vi "FindDeviceNumber.vi"(11 "device":string) -> (3 "device":u16)   [LabVIEW 2022 SP3]
uses:
  Mic/Mic_Global.vi
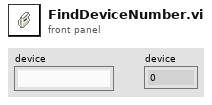
[diagram p1: front panel]
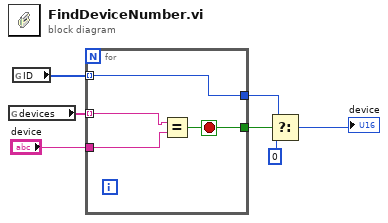
[diagram p0: block diagram]
diagram:
  n1 = global read "Mic_Global.vi" "devices"() -> (w7:string[])
  n2 = global read "Mic_Global.vi" "ID"() -> (w1:i32[])
  n3 = for {
    tunnel: w7 -> [w9] mode=indexing
    tunnel: "device" -> [w11]
    tunnel: [w8] -> w4
    tunnel: [w10] -> w5
    tunnel: w1 -> [w8] mode=indexing
    stop <- w10 stop-if-true
    n4 = Equal?(x=w9, y=w11) -> (x = y?=w10:bool)
  }
  n5 = Select(t=w4, s=w5, f=0) -> (s? t:f=→"device":i32)
